vi "NI 9260 Synchronization 9230 (FPGA).vi"() -> ()   [LabVIEW 2021]
uses:
  <vilib>/LabVIEW Targets/FPGA/cRIO/shared/nicrio_ModuleControls/nicrio_cRIO-9260_DataRatesRing2.ctl
  <vilib>/LabVIEW Targets/FPGA/cRIO/shared/nicrio_ModuleControls/nicrio_cRIO-9230_DataRatesRing2.ctl
  <vilib>/rvi/Emulation/niFpgaGetClockAttributes.vi
  <vilib>/rvi/Emulation/niFpgaSctlEmulationGetInTimedLoop.vi
  <vilib>/rvi/Emulation/niFpgaEmulationReportErrorSimple.vi
  <vilib>/rvi/eio/common/nirviEmuTemplatePropertySet_errors.vi
  <vilib>/rvi/eio/common/nirviEmuTemplateMethod_errors.vi
  <vilib>/rvi/interface/RandomDataEmulation/niFpgaRandomDataHandleErrors.vi
  <vilib>/rvi/Emulation/niFpgaCriticalErrorInLSC.vi
  <vilib>/eio/EIOPropertyNode/EIOPropertyNode.xnode
  <vilib>/eio/EIONode/EIONode.xnode
  <vilib>/rvi/DataTransferAndStorage/Container/XNode/niFpgaContainer.xnode
  <vilib>/rvi/interface/RandomDataEmulation/nirviRandomDataFpgaReadWriteTemplate.vi
  <vilib>/rvi/eio/common/nirviEmuTemplatePropertyGet_errors.vi
  <vilib>/rvi/eio/common/nirviEmuTemplatePropertyGet_noerrors.vi
  <vilib>/rvi/eio/common/nirviEmuTemplatePropertySet_noerrors.vi
panel:
  in  "NI 9230 Data Rate":T1=10 items=["12.800 kS/s (NI 9230)"=10, "11.378 kS/s (NI 9230)"=36, "10.240 kS/s (NI 9230)"=21, "9.309 kS/s (NI 9230)"=44, "8.533 kS/s (NI 9230)"=14, "7.877 kS/s (NI 9230)"=52, "7.314 kS/s (NI 9230)"=29, "6.827 kS/s (NI 9230)"=60, "6.400 kS/s (NI 9230)"=18, "6.024 kS/s (NI 9230)"=68, "5.689 kS/s (NI 9230)"=37, "5.389 kS/s (NI 9230)"=76, "5.120 kS/s (NI 9230)"=22, "4.876 kS/s (NI 9230)"=84, "4.655 kS/s (NI 9230)"=45, "4.452 kS/s (NI 9230)"=92, "4.267 kS/s (NI 9230)"=26, "4.096 kS/s (NI 9230)"=100, "3.938 kS/s (NI 9230)"=53, "3.657 kS/s (NI 9230)"=30, "3.413 kS/s (NI 9230)"=61, "3.200 kS/s (NI 9230)"=34, "3.012 kS/s (NI 9230)"=69, "2.844 kS/s (NI 9230)"=38, "2.695 kS/s (NI 9230)"=77, "2.560 kS/s (NI 9230)"=42, "2.438 kS/s (NI 9230)"=85, "2.327 kS/s (NI 9230)"=46, "2.226 kS/s (NI 9230)"=93, "2.133 kS/s (NI 9230)"=50, "2.048 kS/s (NI 9230)"=101, "1.969 kS/s (NI 9230)"=54, "1.829 kS/s (NI 9230)"=58, "1.707 kS/s (NI 9230)"=62, "1.600 kS/s (NI 9230)"=66, "1.506 kS/s (NI 9230)"=70, "1.422 kS/s (NI 9230)"=74, "1.347 kS/s (NI 9230)"=78, "1.280 kS/s (NI 9230)"=82, "1.219 kS/s (NI 9230)"=86, "1.164 kS/s (NI 9230)"=90, "1.113 kS/s (NI 9230)"=94, "1.067 kS/s (NI 9230)"=98, "1.024 kS/s (NI 9230)"=102, "0.985 kS/s (NI 9230)"=106]
  out "NI 9230 FIFO Time Out":bool
  in  "stop":bool
  out "NI 9260 FIFO Time Out":bool
  in  "NI 9260 Data Rate":T2=1 items=["51.200 kS/s (NI 9260)"=1, "25.600 kS/s (NI 9260)"=2, "17.067 kS/s (NI 9260)"=3, "12.800 kS/s (NI 9260)"=4, "10.240 kS/s (NI 9260)"=5, "8.533 kS/s (NI 9260)"=6, "7.314 kS/s (NI 9260)"=7, "6.400 kS/s (NI 9260)"=8, "5.689 kS/s (NI 9260)"=9, "5.120 kS/s (NI 9260)"=10, "4.654 kS/s (NI 9260)"=11, "4.267 kS/s (NI 9260)"=12, "3.938 kS/s (NI 9260)"=13, "3.657 kS/s (NI 9260)"=14, "3.413 kS/s (NI 9260)"=15, "3.200 kS/s (NI 9260)"=16, "3.012 kS/s (NI 9260)"=17, "2.845 kS/s (NI 9260)"=18, "2.695 kS/s (NI 9260)"=19, "2.560 kS/s (NI 9260)"=20, "2.438 kS/s (NI 9260)"=21, "2.328 kS/s (NI 9260)"=22, "2.226 kS/s (NI 9260)"=23, "2.133 kS/s (NI 9260)"=24, "2.048 kS/s (NI 9260)"=25, "1.969 kS/s (NI 9260)"=26, "1.896 kS/s (NI 9260)"=27, "1.829 kS/s (NI 9260)"=28, "1.765 kS/s (NI 9260)"=29, "1.707 kS/s (NI 9260)"=30, "1.652 kS/s (NI 9260)"=31]
  out "FPGA Error out":errorcluster
  # "Overview: Demonstrates how to synchronize the NI 9260 to the NI 9230.\nRequirements: LabVIEW Full Development System, LV FPGA, and NI RIO\nInstructions: \n1. Run NI 9260 Synchronization (Host).vi"
  # "Output Parameters"
  # "Input Parameters"
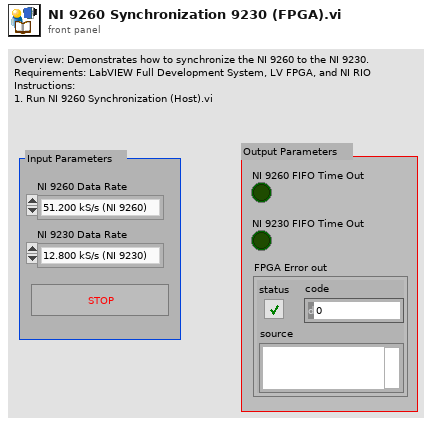
[diagram p1: front panel]
types:
  T1 = typedef "nicrio_cRIO-9230_DataRatesRing2.ctl" = u8
  T2 = typedef "nicrio_cRIO-9260_DataRatesRing2.ctl" = u8
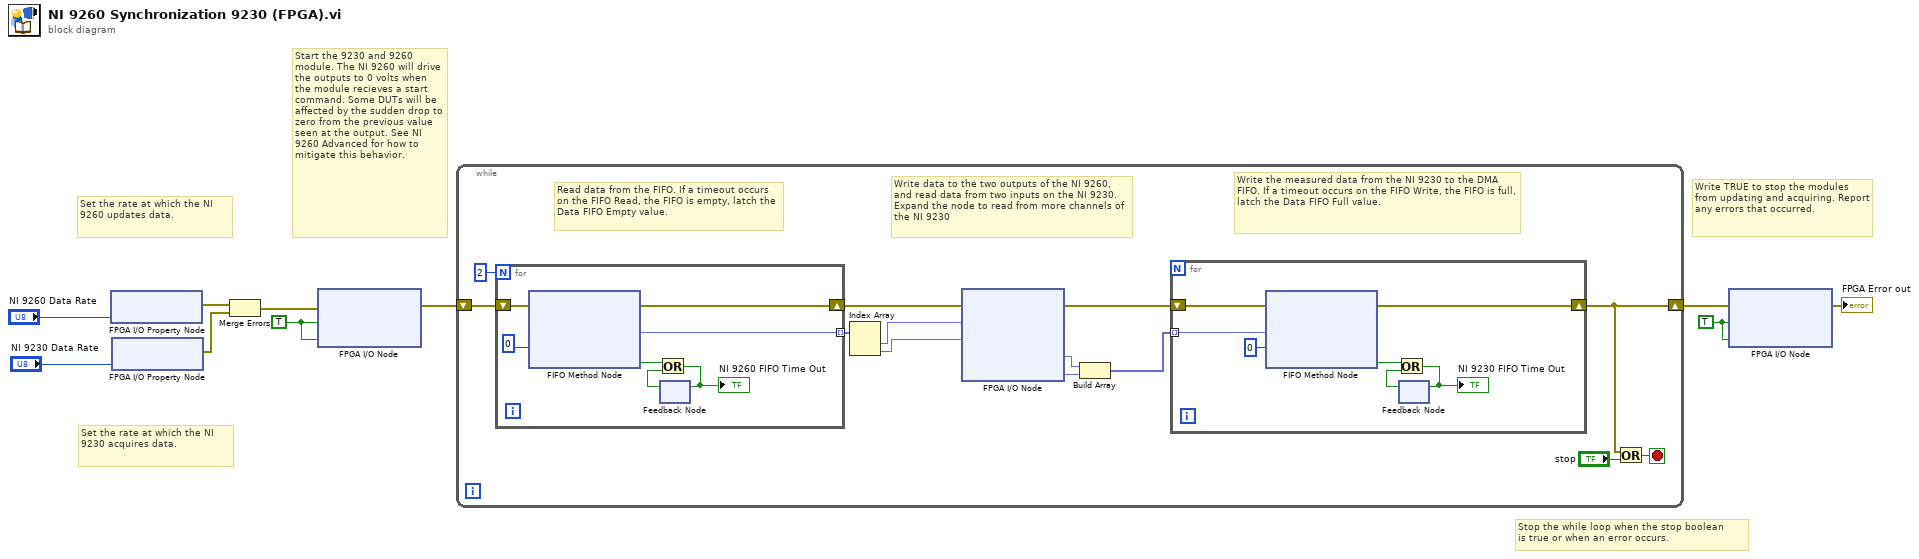
[diagram p0: block diagram]
diagram:
  w5 = TRUE ("Mod1/Stop")
  w6 = TRUE ("Mod1/Start")
  # "Stop the while loop when the stop boolean \nis true or when an error occurs."
  # "Set the rate at which the NI 9230 acquires data."
  # "Write TRUE to stop the modules from updating and acquiring. Report any errors that occurred."
  # "Start the 9230 and 9260 module. The NI 9260 will drive the outputs to 0 volts when the module recieves a start command. Some DUTs will be affected by the sudden drop to zero from the previous value seen at the output. See NI 9260 Advanced for how to mitigate this behavior."
  # "Set the rate at which the NI 9260 updates data."
  n1 = xnode "FPGA I/O Property Node"("Data Rate"="NI 9260 Data Rate") -> ("error out"=w10:errorcluster)  [unwired: 2 in, 1 out]
  n2 = xnode "FPGA I/O Property Node"("Data Rate"="NI 9230 Data Rate") -> ("error out"=w2:errorcluster)  [unwired: 2 in, 1 out]
  n3 = Merge Errors(w10, w2) -> (w3:errorcluster)
  n4 = xnode "FPGA I/O Node"("error in"=w3, "Mod3/Start"=w6, "Mod4/Start"=w6) -> ("error out"=w9:errorcluster)  [unwired: 2 in, 2 out]
  n5 = while {
    shift-right: [w11] -> w8
    shift-left: w9 -> [w23]
    stop <- w21 stop-if-true
    # "Write the measured data from the NI 9230 to the DMA FIFO. If a timeout occurs on the FIFO Write, the FIFO is full, latch the Data FIFO Full value."
    # "Read data from the FIFO. If a timeout occurs on the FIFO Read, the FIFO is empty, latch the Data FIFO Empty value."
    # "Write data to the two outputs of the NI 9260, and read data from two inputs on the NI 9230. Expand the node to read from more channels of the NI 9230"
    n6 = for {
      N: 2 -> [_]
      tunnel: [w31] -> w18 mode=indexing
      shift-right: [w32] -> w22
      shift-left: w23 -> [w33]
      n7 = xnode ("FIFO Method Node")("Timeout"=0, "error in (no error)"=w33) -> ("Element"=w31:fxp<+/-,24,4>, "Timed Out?"=w36:bool, "error out"=w32:errorcluster)  [unwired: 1 in, 1 out]
      n8 = feedback #1() -> (w34:bool)  [unwired: 1 in]
      n9 = Or(x=w36, y=w34) -> (x .or. y?=w35:bool)
      "NI 9260 FIFO Time Out" <- w35
      n10 = feedback-in #1(w35) -> ()
    }
    n11 = Index Array(array=w18) -> (element #1=w17:fxp<+/-,24,4>, element #2=w16:fxp<+/-,24,4>)  [unwired: 2 in]
    n12 = xnode "FPGA I/O Node"("error in"=w22, "Mod4/AO0"=w17, "Mod4/AO1"=w16) -> ("error out"=w12:errorcluster, "Mod3/AI0"=w15:fxp<+/-,24,7>, "Mod3/AI1"=w14:fxp<+/-,24,7>)  [unwired: 4 in, 4 out]
    n13 = Build Array(w15, w14) -> (w13:fxp<+/-,24,7>[])
    n14 = for {
      tunnel: w13 -> [w24] mode=indexing
      shift-right: [w29] -> w11
      shift-left: w12 -> [w28]
      n15 = xnode ("FIFO Method Node")("Element"=w24, "Timeout"=0, "error in (no error)"=w28) -> ("Timed Out?"=w25:bool, "error out"=w29:errorcluster)  [unwired: 1 in, 1 out]
      n16 = feedback #2() -> (w27:bool)  [unwired: 1 in]
      n17 = Or(x=w25, y=w27) -> (x .or. y?=w26:bool)
      "NI 9230 FIFO Time Out" <- w26
      n18 = feedback-in #2(w26) -> ()
    }
    n19 = Or(x=w11, y="stop") -> (x .or. y?=w21:bool)
  }
  n20 = xnode "FPGA I/O Node"("error in"=w8, "Mod3/Stop"=w5, "Mod4/Stop"=w5) -> ("error out"=→"FPGA Error out":errorcluster)  [unwired: 2 in, 2 out]
